vi "squRoot.vi"() -> ()   [LabVIEW 2009]
panel:
  out "result 3":dbl
  in  "number":dbl
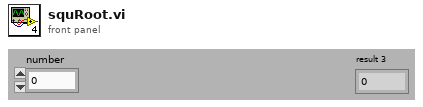
[diagram p1: front panel]
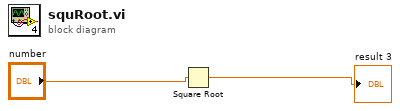
[diagram p0: block diagram]
diagram:
  n1 = Square Root(x="number") -> (sqrt(x)=→"result 3":dbl)
